vi "Events.vi"() -> ()   [LabVIEW 2013]
panel:
  out "Sensors":cluster{"Ultrasonic Distance (In)":dbl}
  out "Auton Variables":cluster{"Hot?":bool}
  out "Shifters":cluster{"Which Gear":bool}
  out "Drive Values":T1
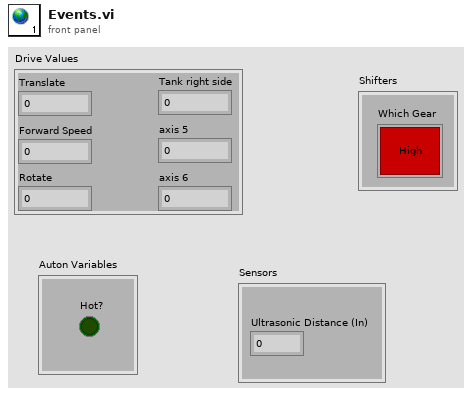
[diagram p1: front panel]
types:
  T1 = cluster{"Translate":dbl, "Forward Speed":dbl, "Rotate":dbl, "Tank right side":dbl, "axis 5":dbl, "axis 6":dbl}
diagram:
